vi "Get Authenticated Athlete.vi"(8 "error in (no error)":errorcluster, 11 "Strava curl in":refnum<class "Strava curl.lvclass">) -> (0 "error out":errorcluster, 2 "Response":string, 3 "Strava curl out":refnum<class "Strava curl.lvclass">)   [LabVIEW 2020, in "Strava curl.lvclass"]
uses:
  Strava curl.lvclass
  Strava curl.lvclass/Strava curl.ctl
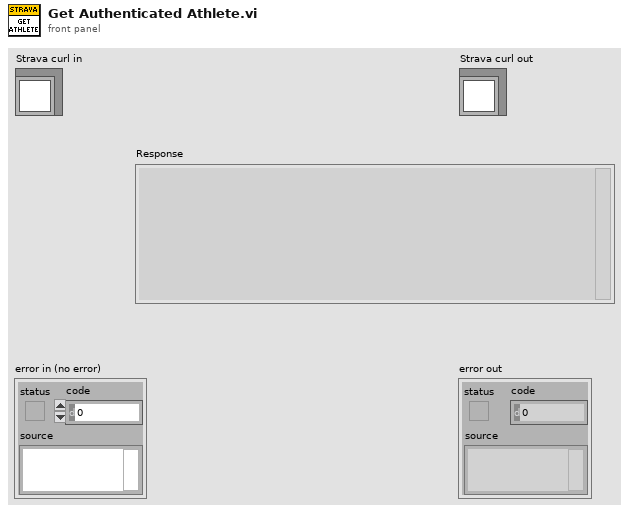
[diagram p1: front panel]
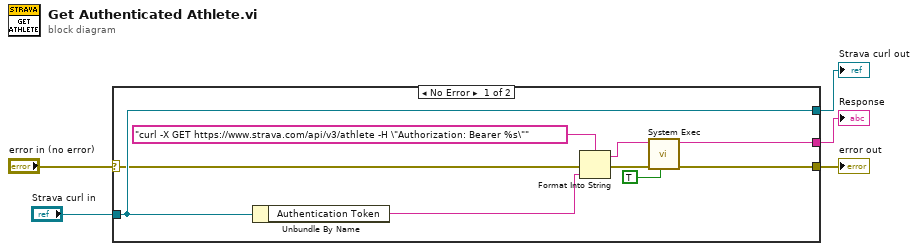
[diagram p0: block diagram]
diagram:
  n1 = case shown="No Error" "error in (no error)" {
    selector: "error in (no error)" -> [w8 w16]
    tunnel: [w9 w16] -> w4
    tunnel: [w14 w15] -> w2
    tunnel: "Strava curl in" -> [w14 w15]
    tunnel: [w6 _] -> w1
    frame No Error {
      n2 = Unbundle By Name(w14) -> ("Authentication Token"=w12:string)
      n3 = Format Into String(format string="curl -X GET https://www.strava.com/api/v3/athlete -H \"Authorization: Bearer %s\"" ("command line"), error in=w8, w12) -> (resulting string=w7:string, error out=w10:errorcluster)  [unwired: 1 in]
      n4 = call <vilib>:"System Exec.vi"("run minimized? (F)"=TRUE, "error in (no error)"=w10, "command line"=w7) -> ("error out"=w9:errorcluster, "standard output"=w6:string)  [unwired: 5 in, 2 out]
    }
    frame Error {
    }
  }
  "error out" <- w4
  "Strava curl out" <- w2
  "Response" <- w1
